vi "Stop Core.vi"(10 "final error code":i32, 11 "Pressure in":refnum<class "Pressure.lvclass">) -> (3 "Pressure out":refnum<class "Pressure.lvclass">)   [LabVIEW 2018, in "Pressure Actor.lvlib" / "Pressure.lvclass"]
doc: "(<B>Filename</B>: Actor Framework.lvlib:Actor.lvclass:Stop Core.vi)\n\nDefines what the actor does before it stops. Use the <B>final error code</B> input to determine whether the actor shut down in response to an error.\n\nBy default, this method passes the Stop message along to all auto-stop nested actors. A descendant class may override this method to define additional behavior, such as shutting down any processes the actor initiated in its override of the Actor Core method."
uses:
  Pressure.lvclass
  <vilib>/ActorFramework/Actor/Actor.lvclass
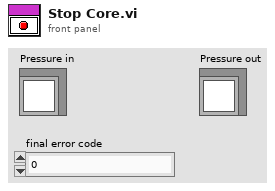
[diagram p1: front panel]
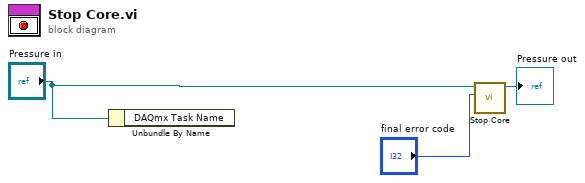
[diagram p0: block diagram]
diagram:
  n1 = Unbundle By Name("Pressure in") -> ()  [unwired: 1 out]
  n2 = call-parent "Stop Core.vi"("final error code"="final error code", "Actor in"="Pressure in") -> ("Actor out"=→"Pressure out":refnum<class "Pressure.lvclass">)  [unwired: 9 in]
